vi "Describe Error.vi"(8 "error in (no error)":errorcluster, 10 "error":errorcluster, 11 "tWorkerCommandRunner in":refnum<class "tWorkerCommandRunner.lvclass">) -> (0 "error out":errorcluster, 3 "tWorkerCommandRunner out":refnum<class "tWorkerCommandRunner.lvclass">)   [LabVIEW 2013, in "tWorkerCommandRunner.lvlib" / "tWorkerCommandRunner.lvclass"]
uses:
  tWorkerCommandRunner.lvclass
  <vilib>/Utility/error.llb/DialogType.ctl
  BSON/tBSONDocument/tBSONDocument.lvclass
  <vilib>/ActorFramework/Actor/Actor.lvclass/Actor.ctl
  tWorkerTCPConnection/msgs/Send Message Msg/Send Message Msg.lvclass/Send Message Msg.ctl
  <vilib>/ActorFramework/Message Enqueuer/Message Enqueuer.lvclass/Message Enqueuer.ctl
  <vilib>/ActorFramework/Message Enqueuer/Enqueue.vi
  BSON/tBSONDocument/addStringElement.vi
  <vilib>/ActorFramework/Message Priority Queue/Priority Enqueue.vi
  tWorkerTCPConnection/msgs/Send Message Msg/Send Message Msg.lvclass
  <vilib>/ActorFramework/Actor/Actor.lvclass
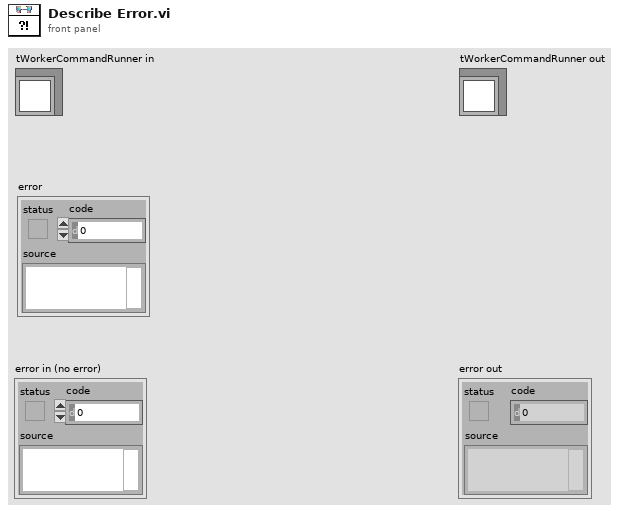
[diagram p1: front panel]
types:
  T1 = typedef "DialogType.ctl" = u16
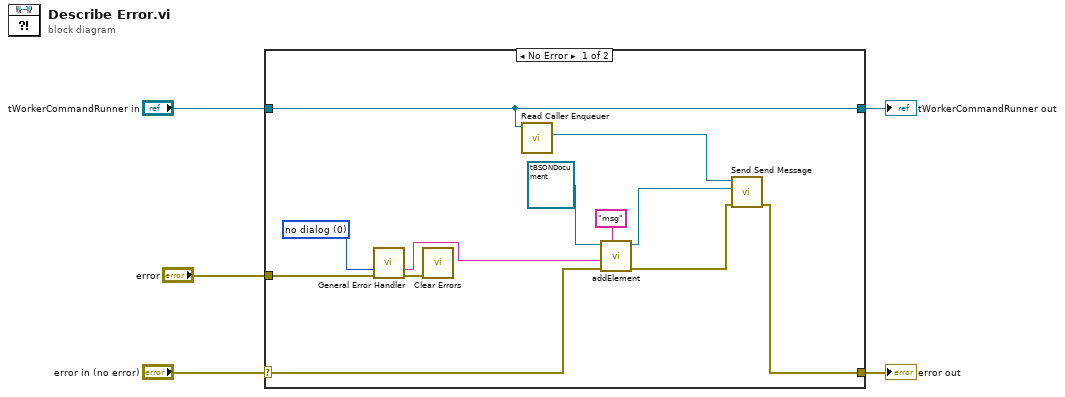
[diagram p0: block diagram]
diagram:
  n1 = case shown="No Error" "error in (no error)" {
    selector: "error in (no error)" -> [w11 w19]
    tunnel: [w6 w19] -> w4
    tunnel: [w15 w18] -> w2
    tunnel: "tWorkerCommandRunner in" -> [w15 w18]
    tunnel: "error" -> [w17 _]
    frame No Error {
      w16 = T1 0 items=["no dialog", "OK message", "continue or stop message", "OK message + warnings", "continue/stop + warnings"] ("type of dialog (OK msg:1)")
      n2 = call <vilib>:"General Error Handler.vi"("type of dialog (OK msg:1)"=w16, "error in (no error)"=w17) -> ("message"=w9:string, "error out"=w10:errorcluster)  [unwired: 9 in, 3 out]
      n3 = call <vilib>:"Clear Errors.vi"("error in (no error)"=w10) -> ()  [unwired: 6 in, 1 out]
      n4 = call <vilib>:"Read Caller Enqueuer.vi"("Actor"=w15) -> ("Caller Enqueuer"=w14:refnum<class "Message Enqueuer.lvclass">)  [unwired: 10 in]
      n5 = call-poly "addElement.vi"("Name"="msg", "error in (no error)"=w11, "Value"=w9, "tBSONDocument in"=refnum<class "tBSONDocument.lvclass"> refnum) -> ("error out"=w7:errorcluster, "tBSONDocument out"=w8:refnum<class "tBSONDocument.lvclass">)  [unwired: 6 in]
      n6 = call "Send Send Message.vi"("error in (no error)"=w7, "Message"=w8, "Message Enqueuer"=w14) -> ("error out"=w6:errorcluster)  [unwired: 7 in, 1 out]
    }
    frame Error {
    }
  }
  "error out" <- w4
  "tWorkerCommandRunner out" <- w2
